vi "Set ROI entry window UI from file-DBL.vi"(8 "error in (no error)":errorcluster, 9 "Keys setup.DBL":T2, 10 "Section name":string, 11 "Refnum in":T1) -> (0 "error out":errorcluster, 3 "Refnum out":T1)   [LabVIEW 2017]
uses:
  Typedefs/Ini file interface (DBL).ctl
  <vilib>/Utility/config.llb/Config Data RefNum.ctl
  User Interface/ROI Entry screen/Globals/gl_ROI Entry UI globals.vi
  <vilib>/Utility/config.llb/NI_LVConfig.lvlib
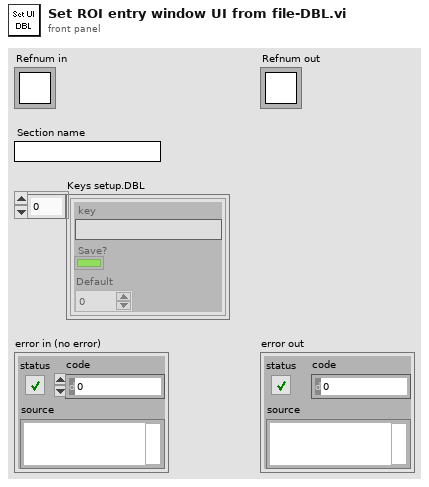
[diagram p1: front panel]
types:
  T1 = typedef "NI_LVConfig.lvlib/Config Data RefNum.ctl" = refnum<k1>
  T2 = typedef "Ini file interface (DBL).ctl" = cluster{"key":string, "Save?":bool, "Default":dbl}[]
  T3 = typedef "ROI entry screen ctrl refs cluster.ctl" = cluster{"Done button":refnum<vi>, "Imaging button":refnum<vi>, "Acquisition button":refnum<vi>, "POI dwell time (us)":refnum<vi>, "Scan dwell time per pixel (us)":refnum<vi>, "# of planes":refnum<vi>, "Zoom Ctrl":refnum<vi>, "Equal size":refnum<vi>, "Channel":refnum<vi>, "Image Display":refnum<vi>, "Z-Plane Selector":refnum<vi>, "Number of lines left":refnum<vi>, "Z-stack folder path":refnum<vi>, "POI Density":refnum<vi>, "Arb Plane Entry":refnum<vi>, "Whole plane":refnum<vi>, "Clear Last":refnum<vi>, "Clear All":refnum<vi>, "Trial Length (sec)":refnum<vi>, "Palette Type":refnum<vi>, "Intensity slider":refnum<vi>, "# POI":refnum<vi>, "Max Z Proj":refnum<vi>, "Zplane ind":refnum<vi>, "Wavelength (nm)":refnum<vi>, "Number of Trials":refnum<vi>, "Funct stim.trig.enable":refnum<vi>, "Funct stim.trig.delay (s)":refnum<vi>, "Line Mode":refnum<vi>, "Step size (µm)":refnum<vi>, "ROI move mode":refnum<vi>, "Cool-down time (s)":refnum<vi>, "Enable cool-down time":refnum<vi>, "Motor Z ind. (um)":refnum<vi>, "AOL Z ind. (um)":refnum<vi>, "Load Reference Image":refnum<vi>}
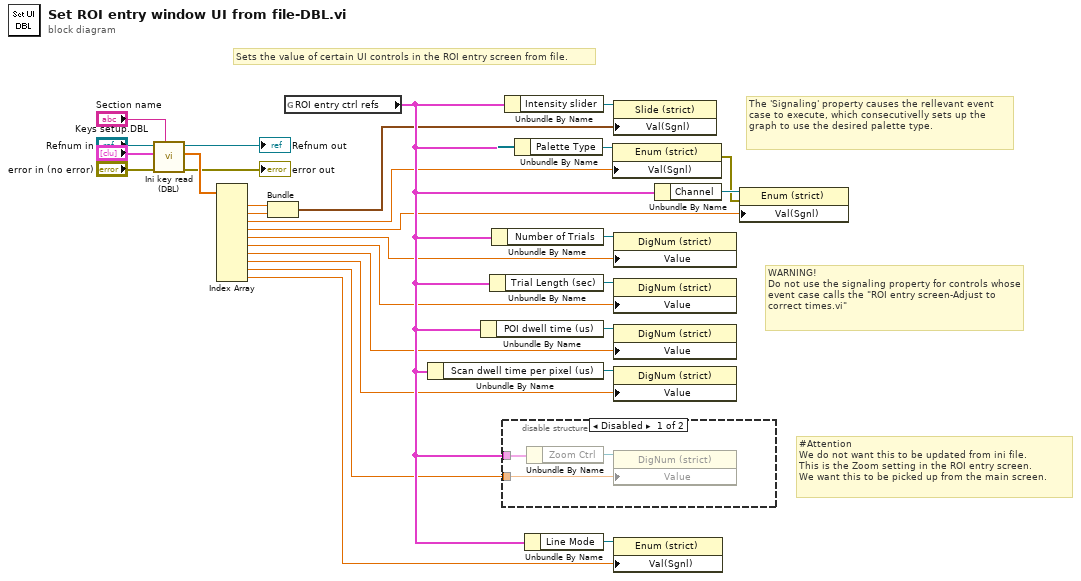
[diagram p0: block diagram]
diagram:
  # "#Attention\nWe do not want this to be updated from ini file.\nThis is the Zoom setting in the ROI entry screen.\nWe want this to be picked up from the main screen."
  # "WARNING!\nDo not use the signaling property for controls whose event case calls the \"ROI entry screen-Adjust to correct times.vi\""
  # "The 'Signaling' property causes the rellevant event case to execute, which consecutivelly sets up the graph to use the desired palette type."
  # "Sets the value of certain UI controls in the ROI entry screen from file."
  n1 = call "Ini key read (DBL).vi"("Section name"="Section name", "error in (no error)"="error in (no error)", "Parameter names & setup"="Keys setup.DBL", "Ini file refnum in"="Refnum in") -> ("error out"=→"error out":errorcluster, "Value read/used"=w26:dbl[], "Ini file refnum out"=→"Refnum out":T1)  [unwired: 5 in]
  n2 = Index Array(array=w26) -> (element #1=w12:dbl, element #2=w11:dbl, element #3=w2:dbl, element #4=w9:dbl, element #5=w8:dbl, element #6=w7:dbl, element #7=w6:dbl, element #8=w5:dbl, element #9=w4:dbl, element #10=w3:dbl)  [unwired: 10 in]
  n3 = Bundle("value"=w12, "value"=w11) -> (w10:cluster{"value":dbl, "value":dbl})  [unwired: 1 in]
  n4 = global read "gl_ROI Entry UI globals.vi" "ROI entry ctrl refs"() -> (w13:T3)
  n5 = Unbundle By Name(w13) -> ("Scan dwell time per pixel (us)"=w14:refnum<vi>)
  n6 = Unbundle By Name(w13) -> ("POI dwell time (us)"=w16:refnum<vi>)
  n7 = Unbundle By Name(w13) -> ("Trial Length (sec)"=w19:refnum<vi>)
  n8 = Unbundle By Name(w13) -> ("Number of Trials"=w18:refnum<vi>)
  n9 = disable-structure shown="Disabled" {
    disable-tunnel: w13 -> [w30 _]
    disable-tunnel: w4 -> [w29 _]
    frame Disabled {
      n10 = Unbundle By Name(w30) -> ("Zoom Ctrl"=w31:refnum<vi>)
      n11 = property class="DigNum (strict)"(reference=w31, "Value"=w29) -> ()  [unwired: 1 in, 2 out]
    }
    frame Enabled {
    }
  }
  n12 = Unbundle By Name(w13) -> ("Intensity slider"=w17:refnum<vi>)
  n13 = Unbundle By Name(w13) -> ("Palette Type"=w21:refnum<vi>)
  n14 = Unbundle By Name(w13) -> ("Line Mode"=w15:refnum<vi>)
  n15 = property class="Enum (strict)"(reference=w21, "Val(Sgnl)"=w2) -> (error out=w1:errorcluster)  [unwired: 1 in, 1 out]
  n16 = property class="Slide (strict)"(reference=w17, "Val(Sgnl)"=w10) -> ()  [unwired: 1 in, 2 out]
  n17 = property class="DigNum (strict)"(reference=w18, "Value"=w8) -> ()  [unwired: 1 in, 2 out]
  n18 = property class="DigNum (strict)"(reference=w19, "Value"=w7) -> ()  [unwired: 1 in, 2 out]
  n19 = property class="DigNum (strict)"(reference=w16, "Value"=w6) -> ()  [unwired: 1 in, 2 out]
  n20 = property class="DigNum (strict)"(reference=w14, "Value"=w5) -> ()  [unwired: 1 in, 2 out]
  n21 = property class="Enum (strict)"(reference=w15, "Val(Sgnl)"=w3) -> ()  [unwired: 1 in, 2 out]
  n22 = Unbundle By Name(w13) -> ("Channel"=w20:refnum<vi>)
  n23 = property class="Enum (strict)"(reference=w20, error in=w1, "Val(Sgnl)"=w9) -> ()  [unwired: 2 out]
